vi "SOFandEOF.vi"(8 "error in (no error)":errorcluster, 11 "ISO 14443 A DOWN in":refnum<class "ISO 14443 A DOWN.lvclass">) -> (0 "error out":errorcluster, 3 "ISO 14443 A DOWN out":refnum<class "ISO 14443 A DOWN.lvclass">, 5 "frame":u8[](array[numeric]))   [LabVIEW 2019, in "ISO 14443 A DOWN.lvclass"]
uses:
  ISO 14443 A DOWN.lvclass
  TypeDef/Store.ctl
  ISO 14443 A DOWN.lvclass/ISO 14443 A DOWN.ctl
  RFID system.lvclass
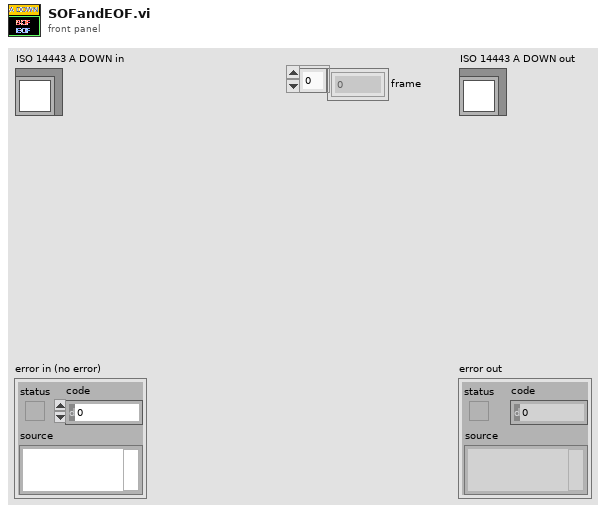
[diagram p1: front panel]
types:
  T1 = typedef "Store.ctl" = enum16{"envelope", "noise", "demSubCar", "CH_frame", "Decode", "demodulate", "in", "out", "sum", "subCarrier", "frame", "command", "encode", "modulate", "encode_UP", "modulate_up", "demod_up", "envelop_up", "sum_up", "out_up", "in_up"}
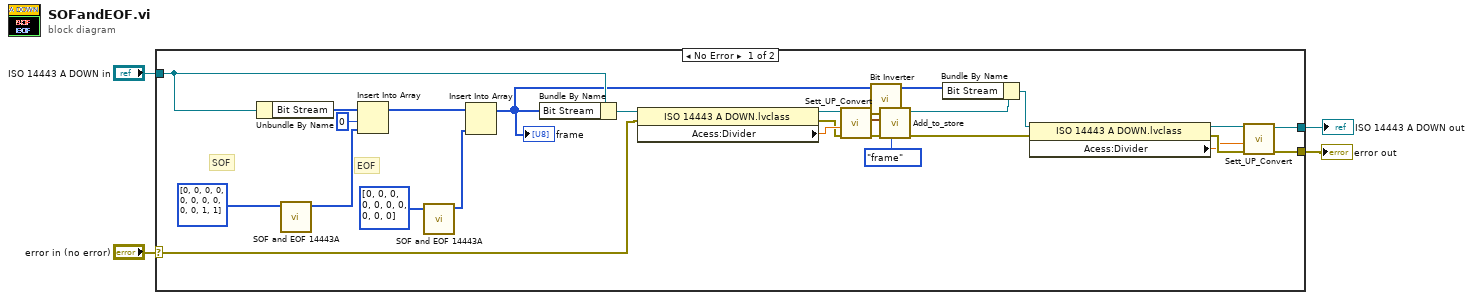
[diagram p0: block diagram]
diagram:
  n1 = case shown="No Error" "error in (no error)" {
    selector: "error in (no error)" -> [w20 w32]
    tunnel: [w11 w33] -> w3
    tunnel: "ISO 14443 A DOWN in" -> [w28 w33]
    tunnel: [w8 w32] -> w2
    frame No Error {
      # "EOF"
      # "SOF"
      n2 = Unbundle By Name(w28) -> ("Bit Stream"=w29:u8[])
      n3 = call "SOF and EOF 14443A.vi"("Bit stream in Miller"=u8[] [0, 0, 0, 0, 0, 0, 0, 0, 0, 0, 1, 1] ("Bit stream out (NRZ encode)")) -> ("Bit stream out Miller"=w17:u8[])  [unwired: 10 in]
      n4 = Insert Into Array(array=w29, index=0, new element=w17) -> (w30:u8[])
      n5 = call "SOF and EOF 14443A.vi"("Bit stream in Miller"=u8[] [0, 0, 0, 0, 0, 0, 0, 0, 0, 0] ("Bit stream out (NRZ encode)")) -> ("Bit stream out Miller"=w15:u8[])  [unwired: 10 in]
      n6 = Insert Into Array(array=w30, new element=w15) -> (w6:u8[])  [unwired: 1 in]
      "frame" <- w6
      n7 = Bundle By Name(cluster=w28, "Bit Stream"=w6) -> (w27:refnum<class "ISO 14443 A DOWN.lvclass">)
      n8 = property class="ISO 14443 A DOWN.lvclass"(reference=w27, error in=w20) -> (reference out=w22:refnum<class "ISO 14443 A DOWN.lvclass">, error out=w19:errorcluster, "Acess:Divider"=w21:dbl)
      n9 = call-dynamic "Sett_UP_Convert.vi"("error in (no error)"=w19, "Divider(1)"=w21, "ISO 14443 A DOWN in"=w22) -> ("error out"=w24:errorcluster, "Waveform"=w25:waveform(dbl), "ISO 14443 A DOWN out"=w26:refnum<class "ISO 14443 A DOWN.lvclass">)  [unwired: 6 in]
      n10 = call "Bit Inverter.vi"("Bit stream in"=w6) -> ("Inverted bit stream out"=w5:u8[])  [unwired: 10 in]
      n11 = call "Add_to_store.vi"("Store"=Store."frame", "error in (no error)"=w24, "Waveform"=w25, "RFID system in"=w26) -> ("error out"=w9:errorcluster, "RFID system out"=w14:refnum<class "ISO 14443 A DOWN.lvclass">)  [unwired: 6 in]
      n12 = Bundle By Name(cluster=w14, "Bit Stream"=w5) -> (w13:refnum<class "ISO 14443 A DOWN.lvclass">)
      n13 = property class="ISO 14443 A DOWN.lvclass"(reference=w13, error in=w9) -> (reference out=w12:refnum<class "ISO 14443 A DOWN.lvclass">, error out=w10:errorcluster, "Acess:Divider"=w7:dbl)
      n14 = call-dynamic "Sett_UP_Convert.vi"("error in (no error)"=w10, "Divider(1)"=w7, "ISO 14443 A DOWN in"=w12) -> ("error out"=w8:errorcluster, "ISO 14443 A DOWN out"=w11:refnum<class "ISO 14443 A DOWN.lvclass">)  [unwired: 6 in, 1 out]
    }
    frame Error {
    }
  }
  "error out" <- w2
  "ISO 14443 A DOWN out" <- w3
